vi "Pusher_Client_CoreMonitor.vi"(8 "ErrIn":errorcluster, 10 "_data":T1, 11 "ClientIn":refnum<class "Client.lvclass">) -> (0 "ErrOut":errorcluster, 3 "Client out":refnum<class "Client.lvclass">)   [LabVIEW 2009, in "Client.lvclass"]
uses:
  Client.lvclass
  public/Pusher_Client_MonitorData.ctl
  Client.lvclass/Client.ctl
  public/Pusher_Client_Global.vi
panel:
  out "Data":string
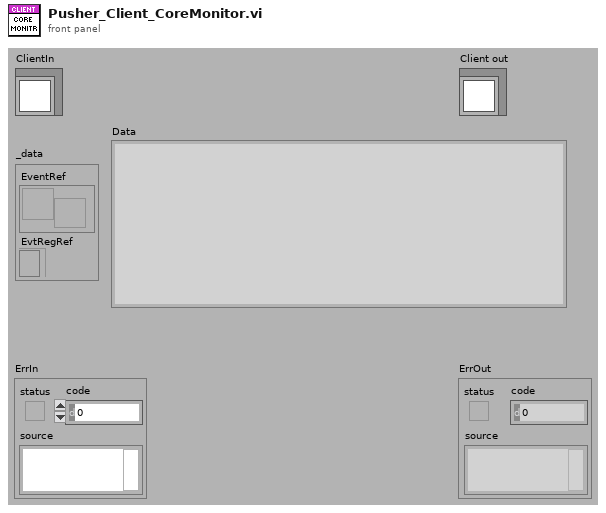
[diagram p1: front panel]
types:
  T1 = typedef "Client.lvclass/Pusher_Client_MonitorData.ctl" = cluster{"EventRef":refnum<user-event>, "EvtRegRef":refnum<event-registration>}
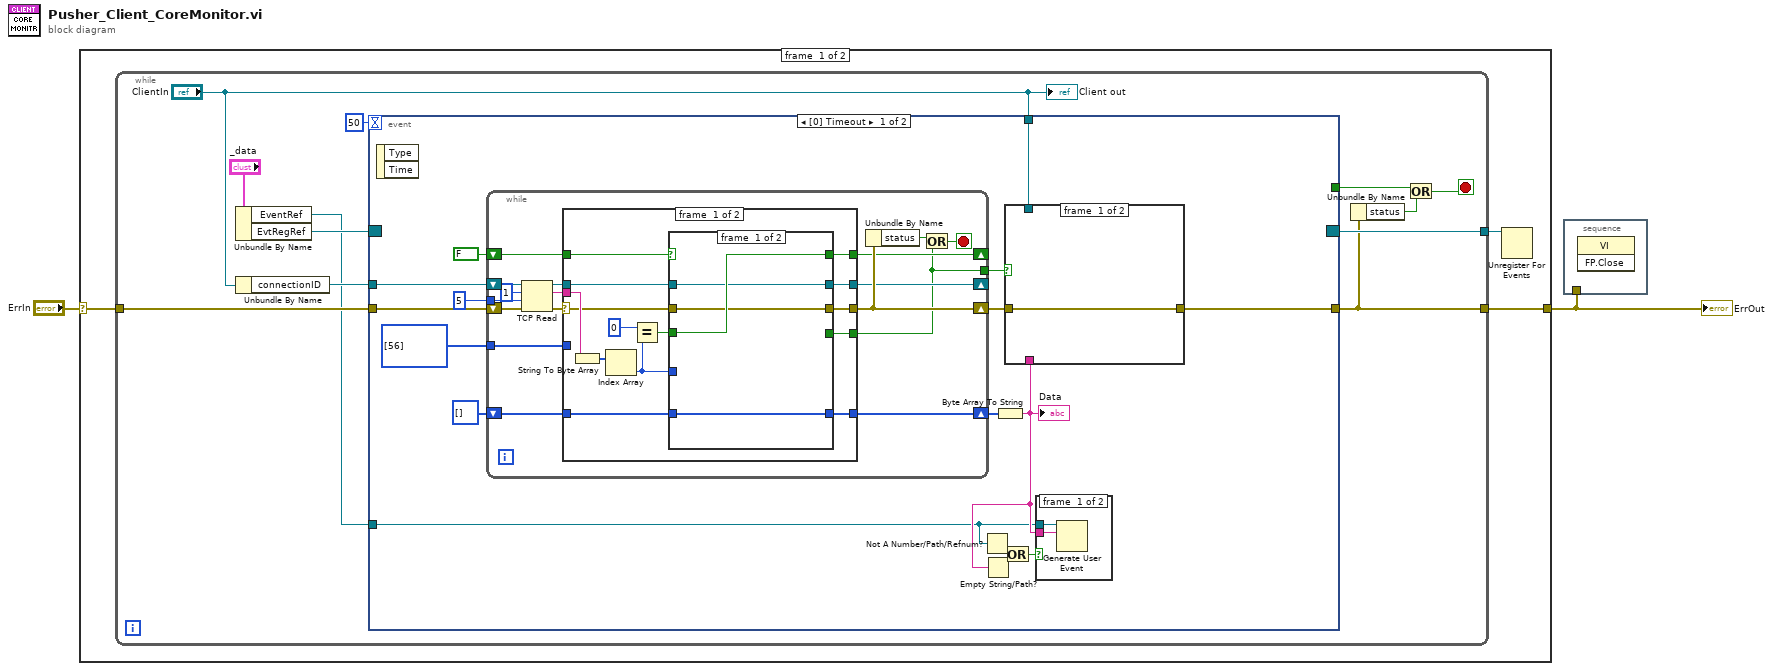
[diagram p0: block diagram]
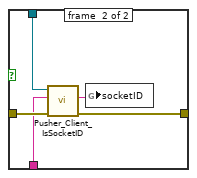
[diagram p2: hidden frame]
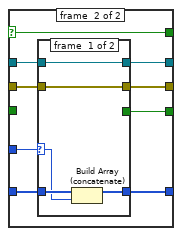
[diagram p4: hidden frame]
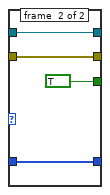
[diagram p5: hidden frame]
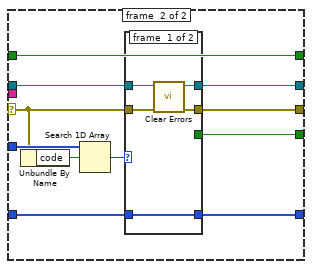
[diagram p6: hidden frame]
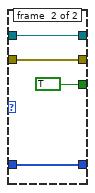
[diagram p7: hidden frame]
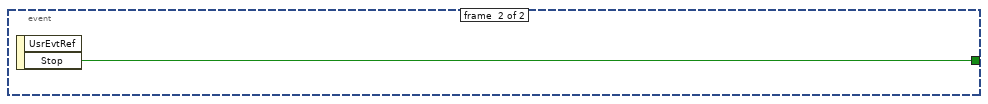
[diagram p8: hidden frame]
diagram:
  n1 = case shown="No Error" "ErrIn" {
    selector: "ErrIn" -> [w5 w115]
    tunnel: [w3 w115] -> w1
    frame #0 {
      n2 = while {
        tunnel: w5 -> [w17]
        tunnel: [w15] -> w4
        tunnel: [w11] -> w3
        stop <- w12 stop-if-true
        n3 = Unbundle By Name("_data") -> ("EventRef"=w7:refnum<user-event>, "EvtRegRef"=w9:refnum<event-registration>)
        n4 = Unbundle By Name("ClientIn") -> ("connectionID"=w8:refnum<k5>)
        n5 = event shown="[0] Timeout" {
          selector: w9 -> [_ _]
          dyn-events: [_ _] -> w15
          timeout: 50 -> [_ _]
          tunnel: w17 -> [w28 _]
          tunnel: w8 -> [w27 _]
          tunnel: [_ w114] -> w13
          tunnel: [w20 _] -> w11
          tunnel: "ClientIn" -> [w21 _]
          tunnel: w7 -> [w18 _]
          event #0 {
            n6 = event-data() -> ()  [unwired: 1 in, 2 out]
            n7 = while {
              tunnel: 5 -> [w55]
              tunnel: i32[] [56] -> [w52]
              shift-right: [w51] -> w23
              shift-left: w28 -> [w57]
              shift-right: [w50] -> _
              shift-left: w27 -> [w58]
              shift-right: [w47] -> w29
              shift-left: u8[] [] -> [w48]
              shift-right: [w43] -> _
              shift-left: FALSE -> [w44]
              tunnel: [w42] -> w19
              stop <- w46 stop-if-true
              n8 = TCP Read(connection ID=w58, bytes to read=1, error in (no error)=w57, 9:w55) -> (connection ID out=w53:refnum<k5>, data out=w49:string, error out=w54:errorcluster)  [unwired: 1 in]
              n9 = case shown="No Error" w54 {
                selector: w54 -> [w66 w102]
                tunnel: w53 -> [w68 w100]
                tunnel: w52 -> [_ w104]
                tunnel: [w65 w101] -> w51
                tunnel: [w67 w99] -> w50
                tunnel: w49 -> [w71 _]
                tunnel: w48 -> [w70 w98]
                tunnel: [w69 w97] -> w47
                tunnel: [w64 w95] -> w42
                tunnel: [w60 w96] -> w43
                tunnel: w44 -> [w61 w96]
                frame #0 {
                  n10 = String To Byte Array(string=w71) -> (unsigned byte array=w72:u8[])
                  n11 = Index Array(array=w72) -> (element=w63:u8)  [unwired: 1 in]
                  n12 = Equal?(x=u8 0, y=w63) -> (x = y?=w59:bool)
                  n13 = case shown="True" w61 {
                    selector: w61 -> [_ w77]
                    tunnel: w63 -> [_ w85]
                    tunnel: w70 -> [w73 w84]
                    tunnel: [w73 w83] -> w69
                    tunnel: w68 -> [w75 w82]
                    tunnel: [w75 w81] -> w67
                    tunnel: w66 -> [w74 w80]
                    tunnel: [w74 w79] -> w65
                    tunnel: [_ w78] -> w64
                    tunnel: [w76 w77] -> w60
                    tunnel: w59 -> [w76 _]
                    frame #0 {
                    }
                    frame #1 {
                      n14 = case shown="255" w85 {
                        selector: w85 -> [w86 _]
                        tunnel: w84 -> [w88 w94]
                        tunnel: [w87 w94] -> w83
                        tunnel: [w90 w93] -> w81
                        tunnel: w82 -> [w90 w93]
                        tunnel: [w89 w92] -> w79
                        tunnel: w80 -> [w89 w92]
                        tunnel: [_ TRUE] -> w78
                        frame #0 {
                          n15 = Build Array (concatenate)(w88, w86) -> (w87:u8[])
                        }
                        frame #1 {
                        }
                      }
                    }
                  }
                }
                frame #1 {
                  n16 = Unbundle By Name(w102) -> ("code"=w105:i32)
                  n17 = Search 1D Array(1D array=w104, element=w105) -> (index of element=w103:i32)  [unwired: 1 in]
                  n18 = case shown="0, Default" w103 {
                    tunnel: w102 -> [w109 w113]
                    tunnel: [w108 w113] -> w101
                    tunnel: [w107 w112] -> w99
                    tunnel: w100 -> [w107 w112]
                    tunnel: [w106 w111] -> w97
                    tunnel: w98 -> [w106 w111]
                    tunnel: [_ TRUE] -> w95
                    frame #0 {
                      n19 = call <vilib>:"Clear Errors.vi"("error in (no error)"=w109) -> ("error out"=w108:errorcluster)  [unwired: 6 in]
                    }
                    frame #1 {
                    }
                  }
                }
              }
              n20 = Unbundle By Name(w51) -> ("status"=w45:bool)
              n21 = Or(x=w45, y=w42) -> (x .or. y?=w46:bool)
            }
            n22 = Not A Number/Path/Refnum?(number/path/refnum=w18) -> (NaN/Path/Refnum?=w26:bool)
            n23 = Byte Array To String(unsigned byte array=w29) -> (string=w22:string)
            "Data" <- w22
            n24 = Empty String/Path?(string/path=w22) -> (empty?=w25:bool)
            n25 = Or(x=w26, y=w25) -> (x .or. y?=w24:bool)
            n26 = case shown="True" w19 {
              tunnel: w23 -> [w34 w39]
              tunnel: w22 -> [_ w38]
              tunnel: w21 -> [_ w37]
              tunnel: [w34 w36] -> w20
              frame #0 {
              }
              frame #1 {
                n27 = call "Pusher_Client_IsSocketID.vi"("ErrIn"=w39, "Frame"=w38, "Client in"=w37) -> ("ErrOut"=w36:errorcluster, "socketID"=w35:string)  [unwired: 5 in, 2 out]
                n28 = global write "Pusher_Client_Global.vi" "socketID"(w35) -> ()
              }
            }
            n29 = case shown="False" w24 {
              tunnel: w22 -> [w41 _]
              tunnel: w18 -> [w40 _]
              frame #0 {
                n30 = Generate User Event(user event=w40, event data cluster=w41) -> ()  [unwired: 1 in, 2 out]
              }
              frame #1 {
              }
            }
          }
          event #1 {
            n31 = event-data() -> ("Stop"=w114:bool)  [unwired: 1 in, 1 out]
          }
        }
        n32 = Unbundle By Name(w11) -> ("status"=w14:bool)
        n33 = Or(x=w13, y=w14) -> (x .or. y?=w12:bool)
        "Client out" <- "ClientIn"
      }
      n34 = Unregister For Events(event registration refnum=w4) -> ()  [unwired: 1 in, 1 out]
    }
    frame #1 {
    }
  }
  "ErrOut" <- w1
  n35 = stacked-sequence {
    tunnel: w1 -> [_]
    frame #0 {
      n36 = invoke class="VI" method="FP.Close"() -> ()  [unwired: 3 in, 3 out]
    }
  }
